vi "Pfeiffer Vacuum MiniTest Current State.vi"(8 "error in (no error)":errorcluster, 10 "Adress of unit":u16=1 min=1 max=999 step=1, 11 "COM Port Name in":refnum<visa-resource-name>="COM1") -> (0 "error out":errorcluster, 1 "State out":u8(ring) items=["Power on"=0, "Power on (wait)"=2, "Wait HV-off stable"=3, "Wait HV-on stable"=4, "Ignition optimization"=5, "Wait for ignition"=6, "Wait for current"=7, "Wait for stable"=8, "Wait for vacuum"=10, "Heating"=20, "Measure"=30, "Error (new)"=100, "Error"=102, "Unrecoverable error (new)"=104, "Unrecoverable error"=106, "SW update"=110], 2 "response (data)":string)   [LabVIEW 2021]
doc: "This VI is an example of how to use the Pfeiffer Vacuum subVIs programmatically. This VI first initializes the instrument, takes measurements, then closes the instrument."
uses:
  <instrlib>/Pfeiffer Vacuum/Pfeiffer Vacuum.lvlib
panel:
  # "Current State (read only)"
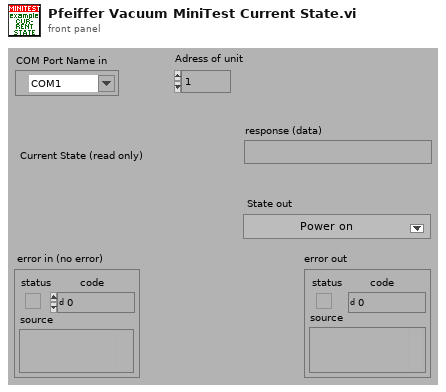
[diagram p1: front panel]
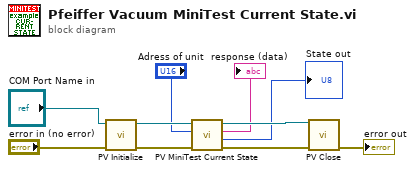
[diagram p0: block diagram]
diagram:
  n1 = call <instrlib>:"PV Initialize.vi"("error in (no error)"="error in (no error)", "VISA session in"="COM Port Name in") -> ("error out"=w10:errorcluster, "VISA session out"=w8:refnum<visa-resource-name>)  [unwired: 8 in]
  n2 = call <instrlib>:"PV MiniTest Current State.vi"("error in (no error)"=w10, "Adress of unit"="Adress of unit", "VISA session"=w8) -> ("error out"=w9:errorcluster, "State out"=→"State out":u8, "response (data) out"=→"response (data)":string, "dup VISA session"=w7:refnum<visa-resource-name>)  [unwired: 5 in]
  n3 = call <instrlib>:"PV Close.vi"("VISA session"=w7, "error in (no error)"=w9) -> ("error out"=→"error out":errorcluster)  [unwired: 13 in]
